vi "AlliGator Clear Phasor Ratio Reference.vi"(8 "error in (no error)":errorcluster, 9 "Reference Number":i32, 10 "State Indicators Refnum":refnum<vi>, 11 "Phasor Graph Refnum":refnum<vi>) -> (0 "Error Out":errorcluster)   [LabVIEW 2021, in "AlliGator Phasor Graph.lvlib"]
doc: "Removes Phasor Graph annotation representing one of the references."
uses:
  AlliGator Phasor Graph.lvlib
  AlliGator State Indicator.ctl
  AlliGator Variables List.ctl
  Phasor/Phasor (g, s).ctl
  AlliGator State Indicators List.ctl
  AlliGator Globals, Variables & Constants.lvlib
  Phasor/Phasor.lvlib
  AlliGator GUI.lvlib
  AlliGator Action Engine.lvlib
panel:
  # "see the AlliGator License on the block diagram (Ctrl+E or Window:Show Block Diagram)"
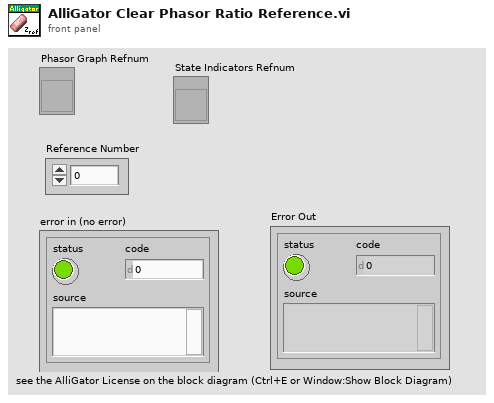
[diagram p1: front panel]
types:
  T1 = typedef "AlliGator Globals, Variables & Constants.lvlib/AlliGator Variables List.ctl" = enum16{"---- GUI ----", "GUI:Initialization Status", "GUI:State Indicators Refnum", "GUI:Original AlliGator Menu Items", "GUI:Current Action Loop State", "GUI:Script in progress", "GUI:Playback", "GUI:Loop Playback", "GUI:Search ROI Used", "GUI:Search ROI", "Decay Graph Max Legend Size", "Intensity Graph Max Legend Size", "Decay Statistics Graph Max Legend Size", "Phasor Graph Max Legend Size", "Phasor Ratio Graph Max Legend Size", "Lifetime Graph Max Legend Size", "---- Files ----", "Files:Export Dataset Frames as Individual Files", "Files:Show Batch Export Help Balloons", "Files:Frames in Dataset", "Files:ptu File Frame Start Indices", "Files:Current Frame in Dataset", "Files:Current Frame Timestamp", "Files:Dataset Loaded", "Files:Dataset Metadata", "Files:Dataset Channel", "Files:Dataset Data Description", "Files:Background Dataset Metadata", "Files:Background Dataset Channel", "Files:Background Dataset Data Description", "Files:Background File Subtraction", "Files:Background File Path", "Files:Background File Pile-up Correction", "Files:Background File Pixel Well Capacity", "Files:Background File Scaling Factor", "Files:Current Dataset Load Settings", "Files:Dataset Path", "Files:ICCD-specific Information", "Files:Macrotime Gate Separation", "------ Python Plugins ------", "Python Plugins:Information", "Python Plugins:Python Session", "Python Plugins:Valid Python Session?", "---- Source Image ----", "Source Image:ROIs", "Source Image:Current ROI", "Source Image:ROI Event Refnum", "X_Source Image Display Range", "X_Source Image Palette Information", "X_Type of Displayed Image", "X_Time Gate Slider", "Source Image:Palette List", "Source Image:Scale", "Source Image:ROI Overlay Color", "Source Image:Overlay to Erase", "Source Image:Is Displayed Image Accumulated", "---- Image Profile Window ----", "Image Profile:Overlay ROI in Source Image", "Image Profile:Window Event Refnum", "Image Profile:IntensityType", "Image Profile:Intensity Average Type", "Image Profile:Intensity-weighted SDV", "Image Profile:Box Profile Type", "Image Profile:Window Open", "Image Profile:Plotted Fit Parameter", "Source Image:White Light Image Modified", "Source Image:Mask Image Modified", "------ Phasor Graph -------", "Phasor Graph:Show Line", "---- Phasor Plot ---", "Phasor Plot:Parameters Changed", "Phasor Plot:FLI Dataset Modified since last Calculation", "Phasor Harmonics Data", "Selected Phasor Harmonics", "Phasor Harmonic Manager Event Refnum", "Phasor Plot:ROIs", "Phasor Plot::Current ROI", "Phasor Plot:ROI Event Refnum", "Phasor Plot:Image Reference Points", "Phasor Plot:Computed", "Phasor Plot:Palette Information", "Phasor Plot:Palette List", "Phasor Ratio Palette Information", "Phasor Ratio Palette List", "Phasor Plot:Image Scale", "Phasor Plot:Image Overlay to Erase", "Phasor Plot:Image Elements to Update", "Current Phasor Plot Calculation Parameters", "Current Phasor Calibration Options", "Phasor Plot::Reset Cumulated Phasor Plot", "Phasor Plot:Reference 1", "Phasor Plot:Lifetime Reference 1", "Phasor Plot:Reference 1 Frequency", "Phasor Plot:Reference 2", "Phasor Plot:Lifetime Reference 2", "Phasor Plot:Reference 2 Frequency", "---- Decay Analysis ----", "Number of Selected Decays to Fit", "LS Fit Results", "LAR Fit Results", "BS Fit Results", "Last Decay Max - Min", "Best Fit Parameters", "Best Fit Parameter Names", "Actual Size X", "Actual Size Y", "Binning X", "Binning Y", "Actual # Gates", "Dataset Number", "Gates to...", "Gates Skipped", "Gates to keep", "Gate Step", "Gate Separation", "Reversed Gates", "Pile-up Correction", "Pixel Well Capacity", "Background Subtracted", "Background Subtraction Method", "Background Definition Range", "Background File (deprecated)", "Number of Dataset Accumulated", "Array of Accumulated Dataset Paths", "Do Averaged Datasets", "Destination File Path", "Process Plot Target", "Use 1/D as Phasor Frequency", "---- Decay Fit Parameter Map -----", "Decay Fit Parameter Map Palette Information", "Decay Fit Parameter Map Palette List", "Local Decay Graph Window Event Refnum", "------- Local Decay Window ---------", "Use normalized IRF for convolution", "----- Miscellaneous ----", "Skippable Dialog Windows Status"}
  T2 = typedef "AlliGator Action Engine.lvlib/AlliGator State Indicators List.ctl" = enum16{"Phasor Calibration Defined", "Phasor Calibration Series Defined", "Phasor Calibration Map Defined", "Phasor Reference 1 Defined", "Phasor Reference 2 Defined", "Lifetime Reference 1 Defined", "Lifetime Reference 2 Defined", "Phasor Calibration Used", "Phasor Calibration Series Used", "Phasor Calibration Map Used", "Dataset Update Needed", "Phasor Plot Update Needed", "Reference/IRF Defined", "Individual IRFs Defined"}
  T3 = typedef "Phasor.lvlib/Phasor (g, s).ctl" = cluster{"g":dbl, "s":dbl}
  T4 = typedef "LVAnnotationListTypeDef.ctl" = cluster{"Name":string, "Color":u32, "Style":u8, "Point Style":u8, "Name Visible":bool, "Allow Drag":bool, "Annotation Mode":u32, "Plot":i32, "Index":i32, "Position":cluster{"X":dbl, "Y":dbl}, "X Scale":u32, "Y Scale":u32, "Show Arrow":bool, "Lock Name":bool, "Plot Area":i32, "Label Offset":cluster{"X":dbl, "Y":dbl}}[]
  T5 = cluster{"Name":string, "Color":u32, "Style":u8, "Point Style":u8, "Name Visible":bool, "Allow Drag":bool, "Annotation Mode":u32, "Plot":i32, "Index":i32, "Position":cluster{"X":dbl, "Y":dbl}, "X Scale":u32, "Y Scale":u32, "Show Arrow":bool, "Lock Name":bool, "Plot Area":i32, "Label Offset":cluster{"X":dbl, "Y":dbl}}
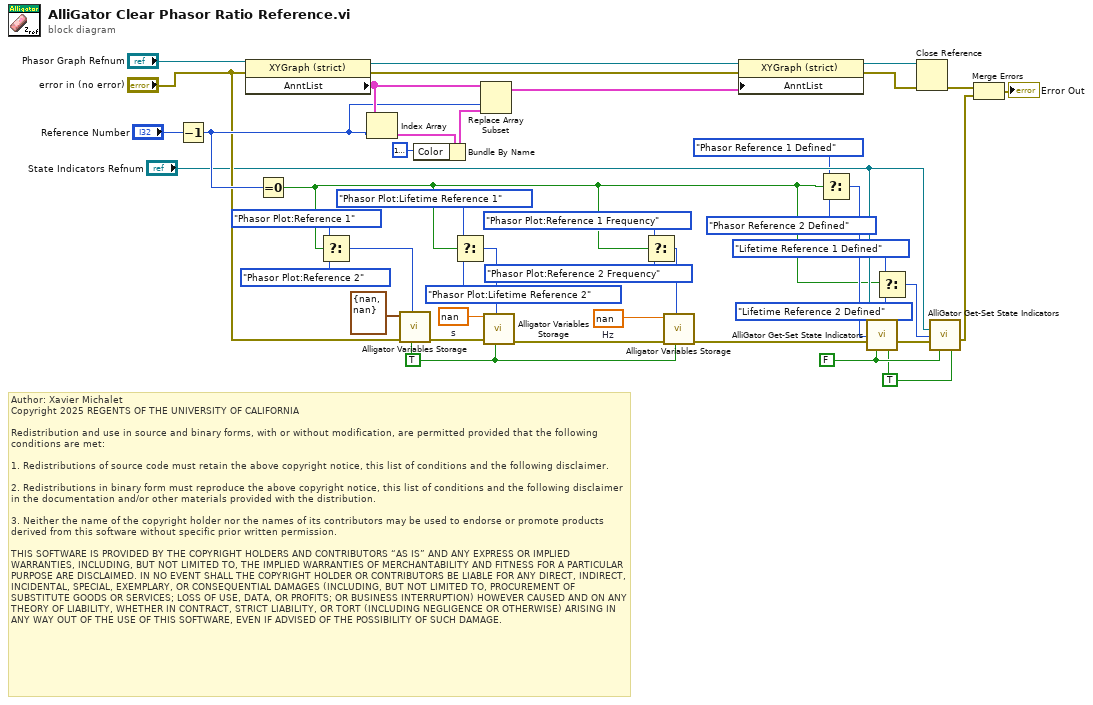
[diagram p0: block diagram]
diagram:
  w1 = TRUE ("Set (T)/Get")
  w2 = dbl[unit] nan  # Hz
  w18 = FALSE ("Set (T)/Unset (F)")
  w21 = dbl[unit] nan  # s
  w7 = TRUE ("Get(F)/Set")
  # "Author: Xavier Michalet\nCopyright 2025 REGENTS OF THE UNIVERSITY OF CALIFORNIA\n\nRedistribution and use in source and binary forms, with or without modification, are permitted provided that the following conditions are met:\n\n1. Redistributions of source code must retain the above copyright notice, this list of conditions and the following disclaimer.\n\n2. Redistributions in binary form must reproduce the above copyright notice, this list of conditions and the following disclaimer in the documentation and/or other materials provided with the distribution.\n\n3. Neither the name of the copyright holder nor the names of its contributors may be used to endorse or promote products derived from this software without specific prior written permission.\n\nTHIS SOFTWARE IS PROVIDED BY THE COPYRIGHT HOLDERS AND CONTRIBUTORS “AS IS” AND ANY EXPRESS OR IMPLIED WARRANTIES, INCLUDING, BUT NOT LIMITED TO, THE IMPLIED WARRANTIES OF MERCHANTABILITY AND FITNESS FOR A PARTICULAR PURPOSE ARE DISCLAIMED. IN NO EVENT SHALL THE COPYRIGHT HOLDER OR CONTRIBUTORS BE LIABLE FOR ANY DIRECT, INDIRECT, INCIDENTAL, SPECIAL, EXEMPLARY, OR CONSEQUENTIAL DAMAGES (INCLUDING, BUT NOT LIMITED TO, PROCUREMENT OF SUBSTITUTE GOODS OR SERVICES; LOSS OF USE, DATA, OR PROFITS; OR BUSINESS INTERRUPTION) HOWEVER CAUSED AND ON ANY THEORY OF LIABILITY, WHETHER IN CONTRACT, STRICT LIABILITY, OR TORT (INCLUDING NEGLIGENCE OR OTHERWISE) ARISING IN ANY WAY OUT OF THE USE OF THIS SOFTWARE, EVEN IF ADVISED OF THE POSSIBILITY OF SUCH DAMAGE."
  n1 = Decrement(x="Reference Number") -> (x-1=w31:i32)
  n2 = property class="XYGraph (strict)"(reference="Phasor Graph Refnum", error in="error in (no error)") -> (reference out=w42:refnum<vi>, error out=w41:errorcluster, "AnntList"=w35:T4)
  n3 = Equal To 0?(x=w31) -> (x = 0?=w4:bool)
  n4 = Select(t=AlliGator_Variables_List."Phasor Plot:Reference 1" ("Alligator Variable"), s=w4, f=AlliGator_Variables_List."Phasor Plot:Reference 2" ("Alligator Variable")) -> (s? t:f=w27:T1)
  n5 = Index Array(array=w35, index=w31) -> (element=w34:T5)
  n6 = call "Alligator Variables Storage.vi"("Get(F)/Set"=w7, "AlliGator Variable"=w27, "Error In"="error in (no error)", "Data in"=T3 {"g"=nan, "s"=nan} ("Phasor Ratio Reference 1")) -> ("Error Out"=w23:errorcluster)  [unwired: 5 in, 2 out]
  n7 = Bundle By Name(cluster=w34, "Color"=u32 16777216) -> (w33:T5)
  n8 = Select(t=AlliGator_Variables_List."Phasor Plot:Lifetime Reference 1" ("Alligator Variable"), s=w4, f=AlliGator_Variables_List."Phasor Plot:Lifetime Reference 2" ("Alligator Variable")) -> (s? t:f=w22:T1)
  n9 = Replace Array Subset(array=w35, new element=w33, index=w31) -> (w40:T4)
  n10 = call "Alligator Variables Storage.vi"("Get(F)/Set"=w7, "AlliGator Variable"=w22, "Error In"=w23, "Data in"=w21) -> ("Error Out"=w9:errorcluster)  [unwired: 5 in, 2 out]
  n11 = Select(t=AlliGator_Variables_List."Phasor Plot:Reference 1 Frequency" ("Alligator Variable"), s=w4, f=AlliGator_Variables_List."Phasor Plot:Reference 2 Frequency" ("Alligator Variable")) -> (s? t:f=w3:T1)
  n12 = call "Alligator Variables Storage.vi"("Get(F)/Set"=w7, "AlliGator Variable"=w3, "Error In"=w9, "Data in"=w2) -> ("Error Out"=w8:errorcluster)  [unwired: 5 in, 2 out]
  n13 = property class="XYGraph (strict)"(reference=w42, error in=w41, "AnntList"=w40) -> (reference out=w39:refnum<vi>, error out=w38:errorcluster)
  n14 = Select(t=AlliGator_State_Indicators_List."Phasor Reference 1 Defined" ("Time-Gated Phasor Analysis Task List"), s=w4, f=AlliGator_State_Indicators_List."Phasor Reference 2 Defined" ("Time-Gated Phasor Analysis Task List")) -> (s? t:f=w15:T2)
  n15 = call "AlliGator Get-Set State Indicators.vi"("State Indicators Refnum"="State Indicators Refnum", "AlliGator State Indicators List"=w15, "Error In"=w8, "ON/OFF"=w18, "Set (T)/Get"=w1) -> ("Error Out"=w20:errorcluster)  [unwired: 8 in, 2 out]
  n16 = Select(t=AlliGator_State_Indicators_List."Lifetime Reference 1 Defined" ("Time-Gated Phasor Analysis Task List"), s=w4, f=AlliGator_State_Indicators_List."Lifetime Reference 2 Defined" ("Time-Gated Phasor Analysis Task List")) -> (s? t:f=w12:T2)
  n17 = Close Reference(reference=w39, error in (no error)=w38) -> (error out=w37:errorcluster)
  n18 = call "AlliGator Get-Set State Indicators.vi"("State Indicators Refnum"="State Indicators Refnum", "AlliGator State Indicators List"=w12, "Error In"=w20, "ON/OFF"=w18, "Set (T)/Get"=w1) -> ("Error Out"=w10:errorcluster)  [unwired: 8 in, 2 out]
  n19 = Merge Errors(w37, w10) -> (→"Error Out":errorcluster)
